vi "camera_mode.vi"() -> ()   [LabVIEW 2021]
uses:
  <vilib>/userDefined/High Color/IMAQdx.ctl
  <vilib>/vision/driver/NI_Vision_Acquisition_Software.lvlib
panel:
  out "Current Mode":u32
  out "Video Modes":T1(array[cluster])
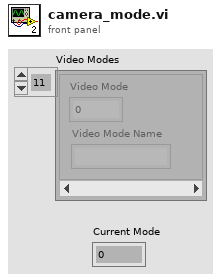
[diagram p1: front panel]
types:
  T1 = cluster{"Video Mode":u32, "Video Mode Name":string}[]
  T2 = typedef "IMAQdx.ctl" = refnum<k21>
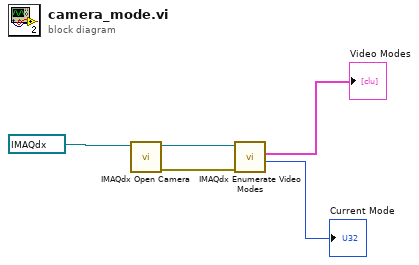
[diagram p0: block diagram]
diagram:
  n1 = call <vilib>:"IMAQdx Open Camera.vi"("Session In"=T2 "cam0") -> ("error out"=w3:errorcluster, "Session Out"=w4:T2)  [unwired: 9 in]
  n2 = call <vilib>:"IMAQdx Enumerate Video Modes.vi"("error in"=w3, "Session In"=w4) -> ("Current Mode"=→"Current Mode":u32, "Video Modes"=→"Video Modes":T1)  [unwired: 6 in, 2 out]
